vi "UDPsender.vi"(6 "receiver's port":u16=61557, 7 "sender's port":u16=61556, 8 "timeout ms":i32=1000, 9 "r-t":bool=TRUE, 10 "Receiver's IP":string="192.168.11.4", 11 "data in":string) -> (0 "error":bool, 3 "r-t time [s]":dbl)   [LabVIEW 2024]
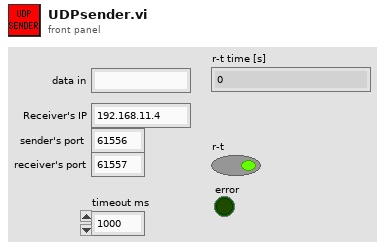
[diagram p1: front panel]
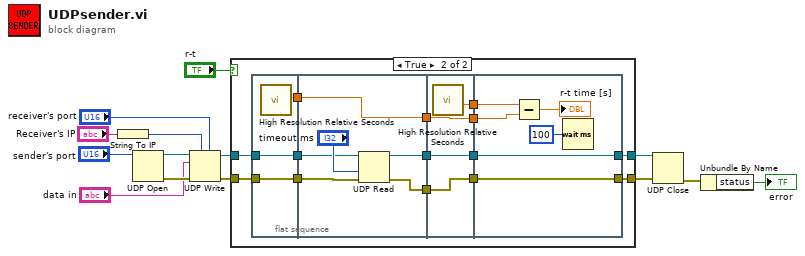
[diagram p0: block diagram]
diagram:
  n1 = String To IP(1:"Receiver's IP") -> (0:w11:u32)
  n2 = UDP Open(11:"sender's port") -> (port=w10:refnum<k16>, 0:w9:errorcluster)  [unwired: 4 in, 1 out]
  n3 = UDP Write(address=w11, port or service name="receiver's port", connection ID=w10, data in="data in", 8:w9) -> (error out=w13:errorcluster, 3:w14:refnum<k16>)  [unwired: 1 in]
  n4 = case shown="True" "r-t" {
    tunnel: w14 -> [w16 w20]
    tunnel: w13 -> [w15 w19]
    tunnel: [w16 w18] -> w8
    tunnel: [w15 w17] -> w7
    frame False {
    }
    frame True {
      n5 = flat-sequence {
        tunnel: w19 -> [w32]
        tunnel: w20 -> [w33]
        tunnel: [w33] -> w30
        tunnel: [w32] -> w29
        tunnel: [w31] -> w28
        tunnel: w30 -> [w36]
        tunnel: [w35] -> w27
        tunnel: w29 -> [w37]
        tunnel: w28 -> [w39]
        tunnel: [w39] -> w26
        tunnel: [w34] -> w25
        tunnel: w27 -> [w43]
        tunnel: [w43] -> w24
        tunnel: [w42] -> w23
        tunnel: [w41] -> w22
        tunnel: w26 -> [w40]
        tunnel: [w40] -> w21
        tunnel: w25 -> [w42]
        tunnel: w24 -> [w45]
        tunnel: w23 -> [w44]
        tunnel: w22 -> [w49]
        tunnel: w21 -> [w48]
        tunnel: [w45] -> w18
        tunnel: [w44] -> w17
        frame #0 {
          n6 = call <vilib>:"High Resolution Relative Seconds.vi"() -> ("relative seconds"=w31:dbl)
        }
        frame #1 {
          n7 = UDP Read(connection ID=w36, timeout ms (25000)="timeout ms", 8:w37) -> (error out=w34:errorcluster, 3:w35:refnum<k16>)  [unwired: 4 out]
        }
        frame #2 {
          n8 = call <vilib>:"High Resolution Relative Seconds.vi"() -> ("relative seconds"=w41:dbl)
        }
        frame #3 {
          n9 = Subtract(x=w49, y=w48) -> (x-y=→"r-t time [s]":dbl)
          n10 = Wait (ms)(milliseconds to wait=u32 100) -> ()  [unwired: 1 out]
        }
      }
    }
  }
  n11 = UDP Close(connection ID=w8, 8:w7) -> (error out=w2:errorcluster)  [unwired: 1 out]
  n12 = Unbundle By Name(w2) -> ("status"=→"error":bool)
